vi "Close Hardware Session.vi"(8 "error in":errorcluster, 10 "card number":u8, 11 "hardware handles":T1) -> (0 "error out":errorcluster)   [LabVIEW 2020, in "AIM ARINC 429 Engine.lvlib" / "Custom Device.lvlib"]
uses:
  Custom Device.lvlib
  Hardware Handles.ctl
  <instrlib>/_AIM 429/Session/Session.lvclass
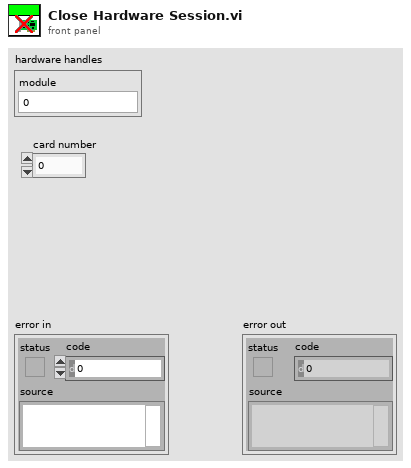
[diagram p1: front panel]
types:
  T1 = typedef "AIM ARINC 429 Engine.lvlib/Custom Device.lvlib/Hardware Handles.ctl" = cluster{"module":u8}
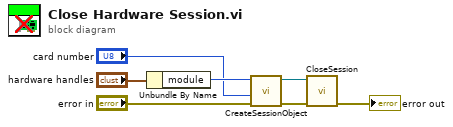
[diagram p0: block diagram]
diagram:
  n1 = Unbundle By Name("hardware handles") -> ("module"=w6:u8)
  n2 = call <instrlib>:"CreateSessionObject.vi"("error in (no error)"="error in", "board id"="card number", "bModuleHandle"=w6) -> ("error out"=w2:errorcluster, "session out"=w5:refnum<class "Session.lvclass">)  [unwired: 7 in]
  n3 = call <instrlib>:"CloseSession.vi"("error in (no error)"=w2, "session in"=w5) -> ("error out"=→"error out":errorcluster)  [unwired: 9 in]
